vi "maxCases.vi"(11 "Loopkennung":u16[](array[numeric])) -> (3 "maxLoop":u8=10)   [LabVIEW 2020, in "PNS.lvlib" / "Komm Modbus.lvlib"]
uses:
  Komm Modbus.lvlib
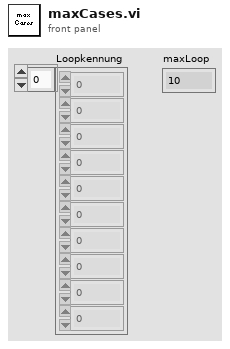
[diagram p1: front panel]
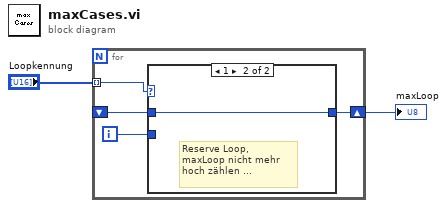
[diagram p0: block diagram]
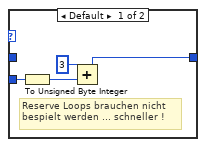
[diagram p2: hidden frame]
diagram:
  n1 = for {
    tunnel: "Loopkennung" -> [w6] mode=indexing
    shift-right: [w4] -> w1
    shift-left: _ -> [w3]
    i -> [w5]
    n2 = case shown="1" w6 {
      tunnel: w5 -> [w10 _]
      tunnel: [w7 w11] -> w4
      tunnel: w3 -> [_ w11]
      frame Default {
        # "Reserve Loops brauchen nicht\nbespielt werden ... schneller !"
        n3 = To Unsigned Byte Integer(number=w10) -> (unsigned 8bit integer=w9:u8)
        n4 = Add(x=u8 3, y=w9) -> (x+y=w7:u8)
      }
      frame 1 {
        # "Reserve Loop,\nmaxLoop nicht mehr \nhoch zählen ..."
      }
    }
  }
  "maxLoop" <- w1
